vi "Command Stopped.vi"(8 "error in (no error)":errorcluster, 9 "Command Name (Instance)":string, 10 "final error code":i32, 11 "Command Processor Actor in":refnum<class "Command Processor Actor.lvclass">) -> (0 "error out":errorcluster, 3 "Command Processor Actor out":refnum<class "Command Processor Actor.lvclass">)   [LabVIEW 2014, in "Robot Actor Framework.lvlib" / "Command Processor Actor.lvlib" / "Command Processor Actor.lvclass"]
uses:
  Command Processor Actor.lvclass
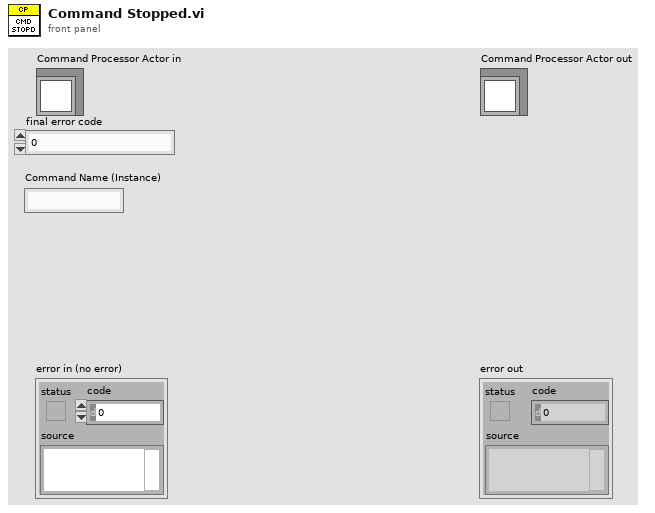
[diagram p1: front panel]
types:
  T1 = enum16{"Critical", "Error", "Warning", "Informational", "Debug"}
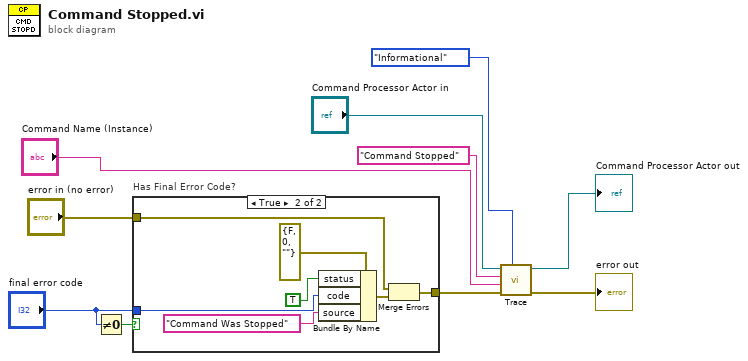
[diagram p0: block diagram]
diagram:
  n1 = Not Equal To 0?(x="final error code") -> (x != 0?=w8:bool)
  n2 = case "Has Final Error Code?" shown="True" w8 {
    tunnel: "error in (no error)" -> [w11 w16]
    tunnel: [w11 w18] -> w6
    tunnel: "final error code" -> [_ w12]
    frame False {
    }
    frame True {
      n3 = Bundle By Name(cluster=errorcluster {"status"=FALSE, "code"=0, "source"=""} ("error constant"), "status"=TRUE, "code"=w12, "source"="Command Was Stopped") -> (w15:errorcluster)
      n4 = Merge Errors(w16, w15) -> (w18:errorcluster)
    }
  }
  n5 = call-dynamic "Trace.vi"("Trace Level"=T1."Informational", "error in (no error)"=w6, "Command Processor Message"="Command Name (Instance)", "Command Processor Action"="Command Stopped", "Command Processor Actor in"="Command Processor Actor in") -> ("error out"=→"error out":errorcluster, "Command Processor Actor out"=→"Command Processor Actor out":refnum<class "Command Processor Actor.lvclass">)  [unwired: 5 in]
